vi "FTW-Endpoint-Multipart-Send.vi"(0 "FTW Endpoint":refnum<class "FTW-Endpoint-TCP.lvclass">, 5 "Multipart Message":string[](array[string]), 7 "Timeout":i32 format="%dmsec", 11 "error in":errorcluster) -> (4 "FTW Endpoint out":refnum<class "FTW-Endpoint-TCP.lvclass">, 6 "Timed out?":bool, 15 "error out":errorcluster)   [LabVIEW 2013, in "FTW-Endpoint-TCP.lvclass"]
uses:
  FTW-Endpoint-TCP.lvclass
  FTW-Endpoint-TCP.lvclass/FTW-Endpoint-TCP.ctl
  Core/src/Error/FTW-ERR-Clear.vi
panel:
  # "Inputs"
  # "Outputs"
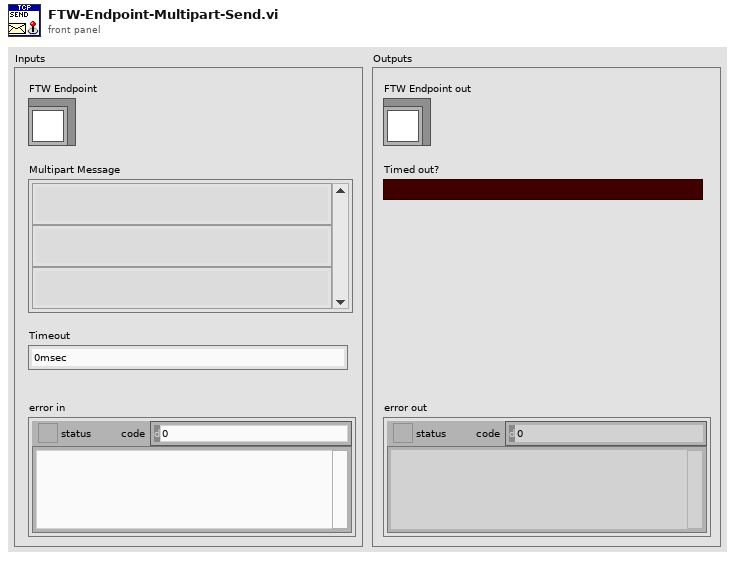
[diagram p1: front panel]
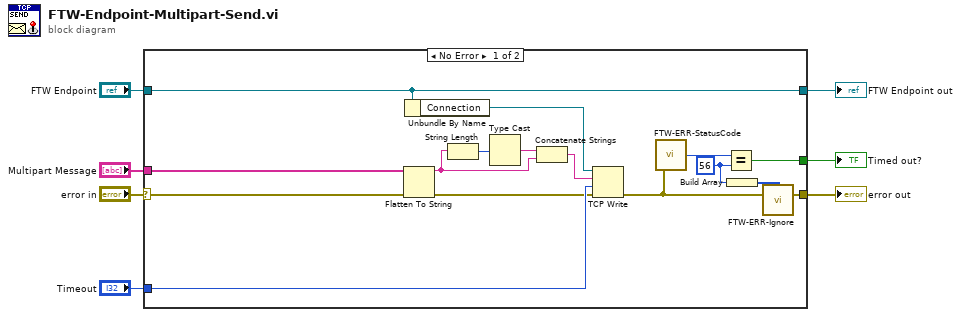
[diagram p0: block diagram]
diagram:
  n1 = case shown="No Error" "error in" {
    selector: "error in" -> [w21 w25]
    tunnel: [w9 w25] -> w7
    tunnel: [w22 w24] -> w5
    tunnel: "FTW Endpoint" -> [w22 w24]
    tunnel: "Multipart Message" -> [w20 _]
    tunnel: [w8 _] -> w2
    tunnel: "Timeout" -> [w23 _]
    frame No Error {
      w12 = 56 ("x")
      n2 = Flatten To String(anything=w20, error in (no error)=w21) -> (data string=w14:string, error out=w19:errorcluster)  [unwired: 2 in, 1 out]
      n3 = Unbundle By Name(w22) -> ("Connection"=w18:refnum<k5>)
      n4 = String Length(string=w14) -> (length=w17:i32)
      n5 = Type Cast(x=w17) -> (*(type *) &x=w16:string)  [unwired: 1 in]
      n6 = Concatenate Strings(w16, w14) -> (w15:string)
      n7 = TCP Write(connection ID=w18, data in=w15, error in (no error)=w19, 9:w23) -> (error out=w10:errorcluster)  [unwired: 2 out]
      n8 = call "FTW-ERR-StatusCode.vi"("error to check"=w10) -> ("Code"=w13:i32)
      n9 = Equal?(x=w13, y=w12) -> (x = y?=w8:bool)
      n10 = Build Array(w12) -> (w11:i32[])
      n11 = call "FTW-ERR-Ignore.vi"("Codes to filter"=w11, "error to filter"=w10) -> ("filtered error"=w9:errorcluster)  [unwired: 13 in]
    }
    frame Error {
    }
  }
  "error out" <- w7
  "FTW Endpoint out" <- w5
  "Timed out?" <- w2
